vi "Save Scan.vi"(8 "error in (no error)":errorcluster, 9 "File IO.lvclass":refnum<class "File IO.lvclass">, 10 "Reader.lvclass":refnum<class "Reader.lvclass">, 11 "Scanner.lvclass":refnum<class "Scanner.lvclass">) -> (0 "error out":errorcluster)   [LabVIEW 2017, in "File IO.lvclass"]
uses:
  File IO.lvclass
  Scanners/Scanner/Scanner.lvclass
  Readers/Reader/Reader.lvclass
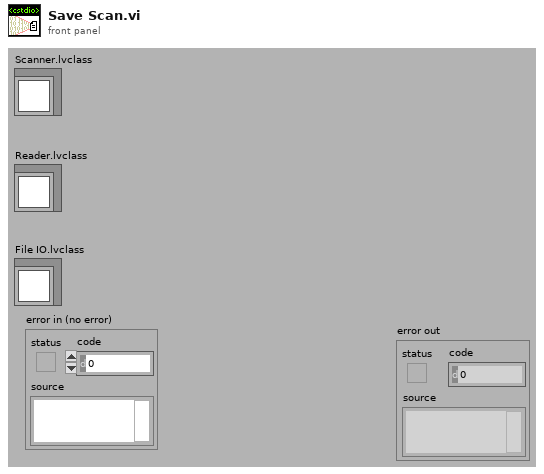
[diagram p1: front panel]
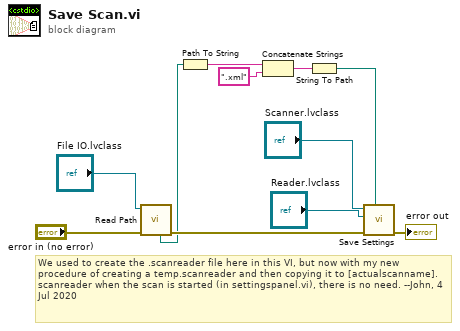
[diagram p0: block diagram]
diagram:
  # "We used to create the .scanreader file here in this VI, but now with my new procedure of creating a temp.scanreader and then copying it to [actualscanname].scanreader when the scan is started (in settingspanel.vi), there is no need. --John, 4 Jul 2020"
  n1 = call-dynamic "Read Path.vi"("error in (no error)"="error in (no error)", "File IO.lvclass in"="File IO.lvclass") -> ("error out"=w7:errorcluster, "Settings Path"=w5:path)  [unwired: 5 in, 3 out]
  n2 = Path To String(path=w5) -> (string=w4:string)
  n3 = Concatenate Strings(w4, ".xml" ("string")) -> (w2:string)
  n4 = String To Path(string=w2) -> (path=w1:path)
  n5 = call "Save Settings.vi"("XML File Path"=w1, "error in (no error)"=w7, "Reader Object"="Reader.lvclass", "Scanner Object"="Scanner.lvclass") -> ("error out"=→"error out":errorcluster)  [unwired: 7 in]
